vi "Set Exposure Mode.vi"(8 "error in (no error)":errorcluster, 10 "Exposure Mode":T1, 11 "Camera in":refnum<class "Camera.lvclass">) -> (0 "error out":errorcluster, 3 "Camera":refnum<class "Camera.lvclass">)   [LabVIEW 2020, in "Camera.lvclass"]
uses:
  Camera.lvclass
  Exposure Mode.ctl
  Camera.lvclass/Camera.ctl
  bin/gindustrialcam_32-1.dll
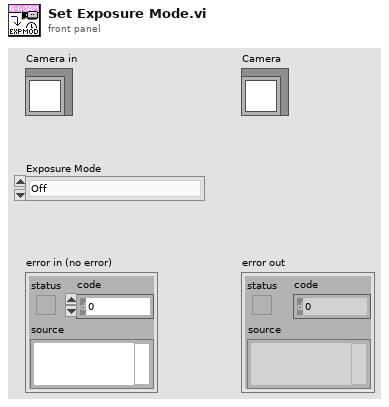
[diagram p1: front panel]
types:
  T1 = typedef "Camera.lvclass/Exposure Mode.ctl" = enum8{"Off", "Timed", "Trigger Width", "Trigger Controller"}
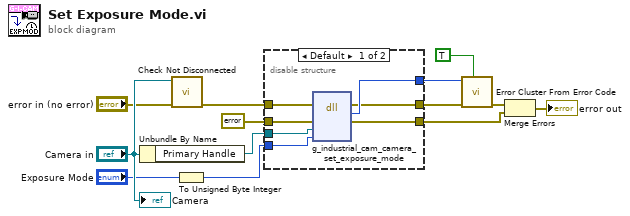
[diagram p0: block diagram]
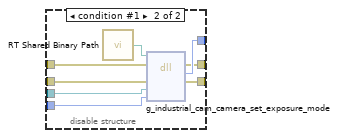
[diagram p2: hidden frame]
diagram:
  n1 = Unbundle By Name("Camera in") -> ("Primary Handle"=w7:refnum<data-value>)
  n2 = call "Check Not Disconnected.vi"("error in (no error)"="error in (no error)", "Camera in"="Camera in") -> ("error out"=w9:errorcluster)  [unwired: 9 in]
  n3 = To Unsigned Byte Integer(number="Exposure Mode") -> (unsigned 8bit integer=w8:u8)
  n4 = disable-structure shown="Default" {
    disable-tunnel: w9 -> [w20 w28]
    disable-tunnel: w8 -> [w19 w27]
    disable-tunnel: w7 -> [w18 w26]
    disable-tunnel: errorcluster {"status"=FALSE, "code"=0, "source"=""} ("error constant") -> [w17 w25]
    disable-tunnel: [w16 w24] -> w4
    disable-tunnel: [w15 w23] -> w2
    disable-tunnel: [w14 w22] -> w1
    frame condition #0 (active) {
      n5 = dll-call lib="C:/serenial/lib/g-industrial-camera/LabVIEW/g_industrial_cam/bin/gindustrialcam_*-1.*" fn="g_industrial_cam_camera_set_exposure_mode"(error in=w20, "err"=w17, "edvr"=w18, "mode"=w19) -> (error out=w14:errorcluster, "Mg_Error"=w15:i32, "err"=w16:errorcluster)  [unwired: 4 in, 1 out]
    }
    frame condition #1 {
      n6 = call "RT Shared Binary Path.vi"() -> ("Path"=w21:path)
      n7 = dll-call lib="C:/serenial/lib/g-industrial-camera/LabVIEW/g_industrial_cam/bin/gindustrialcam_*-1.*" fn="g_industrial_cam_camera_set_exposure_mode"(path in=w21, error in=w28, "err"=w25, "edvr"=w26, "mode"=w27) -> (error out=w22:errorcluster, "Mg_Error"=w23:i32, "err"=w24:errorcluster)  [unwired: 3 in, 1 out]
    }
  }
  n8 = call <vilib>:"Error Cluster From Error Code.vi"("show call chain? (False)"=TRUE, "error in (no error)"=w1, "error code (0)"=w2) -> ("error out"=w3:errorcluster)  [unwired: 6 in]
  n9 = Merge Errors(w3, w4) -> (→"error out":errorcluster)
  "Camera" <- "Camera in"
